vi "Create Empty Temp Folder.vi"(8 "error in (no error)":errorcluster, 11 "Folder Name":string) -> (0 "error out":errorcluster, 3 "Empty Temp Folder":path)   [LabVIEW 2023]
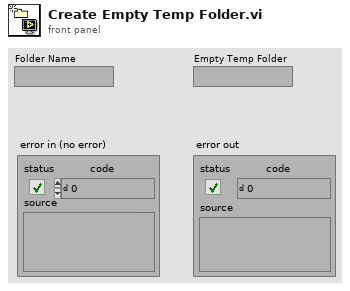
[diagram p1: front panel]
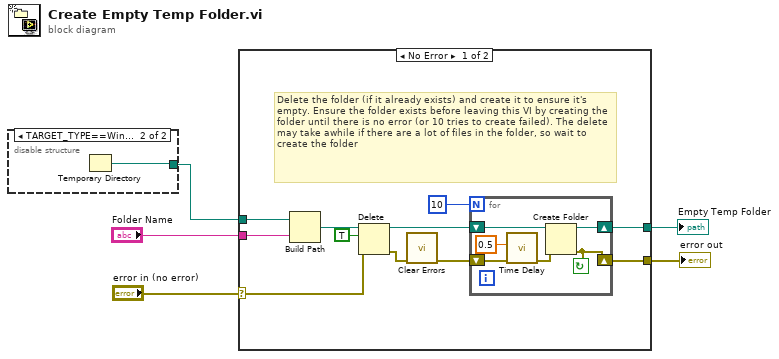
[diagram p0: block diagram]
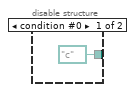
[diagram p3: hidden frame]
diagram:
  n1 = disable-structure shown="TARGET_TYPE==Windows" {
    disable-tunnel: [path "c:/" ("path") w7] -> w5
    frame condition #0 {
    }
    frame condition #1 (active) {
      n2 = Temporary Directory() -> (w7:path)
    }
  }
  n3 = case shown="No Error" "error in (no error)" {
    selector: "error in (no error)" -> [w9 w25]
    tunnel: w5 -> [w18 _]
    tunnel: [w11 _] -> w4
    tunnel: "Folder Name" -> [w10 _]
    tunnel: [w8 w25] -> w1
    frame No Error {
      # "Delete the folder (if it already exists) and create it to ensure it's empty. Ensure the folder exists before leaving this VI by creating the folder until there is no error (or 10 tries to create failed). The delete may take awhile if there are a lot of files in the folder, so wait to create the folder"
      n4 = Build Path(base path=w18, name or relative path=w10) -> (appended path=w16:path)
      n5 = Delete(path (use dialog)=w16, entire hierarchy (F)=TRUE, error in=w9) -> (deleted path=w15:path, error out=w14:errorcluster)  [unwired: 2 in, 1 out]
      n6 = call <vilib>:"Clear Errors.vi"("error in (no error)"=w14) -> ("error out"=w13:errorcluster)  [unwired: 5 in, 1 out]
      n7 = for {
        N: 10 -> [_]
        shift-right: [w23] -> w11
        shift-left: w15 -> [w24]
        shift-right: [w22] -> w8
        shift-left: w13 -> [w21]
        stop <- w22 continue-if-true
        n8 = call "Time Delay"("error in (no error)"=w21, "Delay Time (s)"=0.5) -> ("error out"=w20:errorcluster)  [unwired: 9 in]
        n9 = Create Folder(path (use dialog)=w24, error in=w20) -> (created path=w23:path, error out=w22:errorcluster)  [unwired: 2 out]
      }
    }
    frame Error {
    }
  }
  "Empty Temp Folder" <- w4
  "error out" <- w1
